vi "Image Zoom.vi"(10 "Picture to Insert":picture, 11 "Draw Area Size":T1) -> (2 "Zoom Factor":dbl, 3 "new picture":picture)   [LabVIEW 2016]
uses:
  <vilib>/Utility/miscctls.llb/LVBoundsTypeDef.ctl
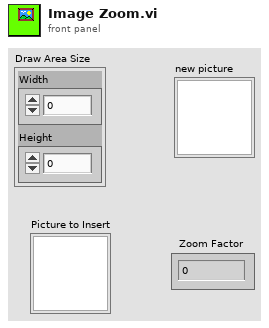
[diagram p1: front panel]
types:
  T1 = typedef "LVBoundsTypeDef.ctl" = cluster{"Width":u32, "Height":u32}
  T2 = typedef "imagedata.ctl" = cluster{"image type":i32, "image depth":i32, "image":u8[], "mask":u8[], "colors":u32[], "Rectangle":cluster{"left":i16, "top":i16, "right":i16, "bottom":i16}}
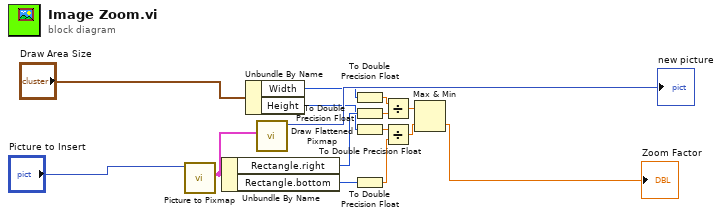
[diagram p0: block diagram]
diagram:
  n1 = call <vilib>:"Picture to Pixmap.vi"("picture"="Picture to Insert") -> ("image data"=w1:T2)  [unwired: 9 in, 1 out]
  n2 = Unbundle By Name(w1) -> ("Rectangle.right"=w11:i16, "Rectangle.bottom"=w9:i16)
  n3 = Unbundle By Name("Draw Area Size") -> ("Width"=w5:u32, "Height"=w7:u32)
  n4 = call <vilib>:"Draw Flattened Pixmap.vi"("image data"=w1) -> ("new picture"=→"new picture":picture)  [unwired: 8 in]
  n5 = To Double Precision Float(number=w5) -> (double precision float=w6:dbl)
  n6 = To Double Precision Float(number=w11) -> (double precision float=w12:dbl)
  n7 = To Double Precision Float(number=w7) -> (double precision float=w8:dbl)
  n8 = To Double Precision Float(number=w9) -> (double precision float=w10:dbl)
  n9 = Divide(x=w6, y=w12) -> (x/y=w4:dbl)
  n10 = Divide(x=w8, y=w10) -> (x/y=w13:dbl)
  n11 = Max & Min(x=w4, y=w13) -> (min(x,y)=→"Zoom Factor":dbl)  [unwired: 1 out]
